vi "Get IBEE Results.vi"(8 "error in (no error)":errorcluster, 11 "niDTS BT INSTR TX in":refnum<class "niDTS BT INSTR TX.lvclass">) -> (0 "error out":errorcluster, 2 "IBE Results":T1, 3 "niDTS BT INSTR TX out":refnum<class "niDTS BT INSTR TX.lvclass">)   [LabVIEW 2015, in "niDTS BT.lvlib" / "niDTS BT INSTR TX.lvclass"]
uses:
  niDTS BT INSTR TX.lvclass
  Tests/Tx Test/Includes/niDTS BT Tx Test INC IBE Results.ctl
  niDTS BT INSTR TX.lvclass/niDTS BT INSTR TX.ctl
  RiviInstDriver/niRfsaBT/Objects/niRfsaBt.lvclass
  niDTS BT.lvlib
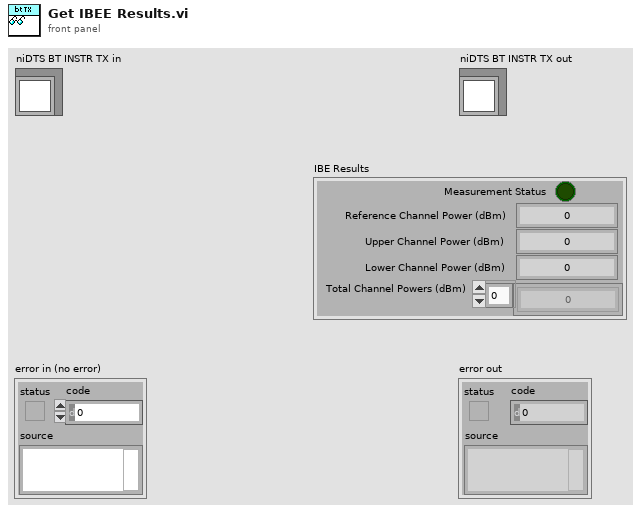
[diagram p1: front panel]
types:
  T1 = typedef "niDTS BT.lvlib/niDTS BT Tx Test INC IBE Results.ctl" = cluster{"Measurement Status":bool, "Reference Channel Power (dBm)":dbl, "Upper Channel Power (dBm)":dbl, "Lower Channel Power (dBm)":dbl, "Total Channel Powers (dBm)":dbl[]}
  T2 = cluster{"MeasurementStatus":enum16{"PASS", "FAIL"}, "ReferenceChannelPower":dbl, "UpperChannelTotalPower":dbl, "LowerChannelTotalPower":dbl, "TotalChannelPower":dbl[]}
  T3 = typedef "niRfsaBT.lvclass/niRfsaBT INC Handle.ctl" = refnum<data-value>
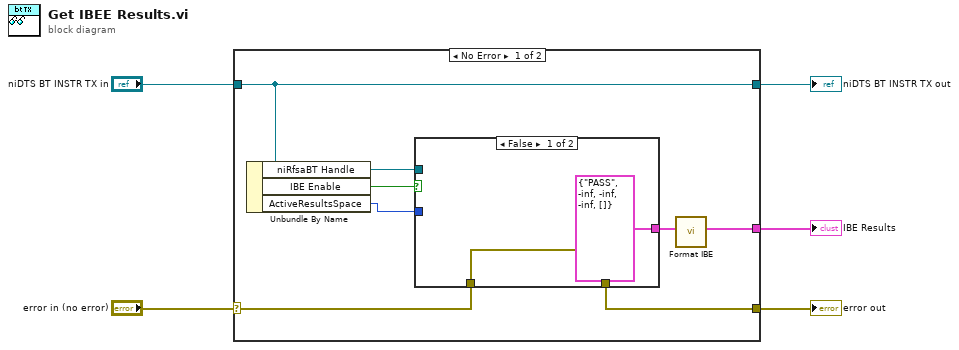
[diagram p0: block diagram]
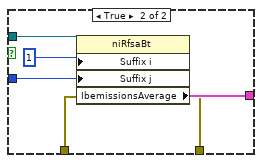
[diagram p2: hidden frame]
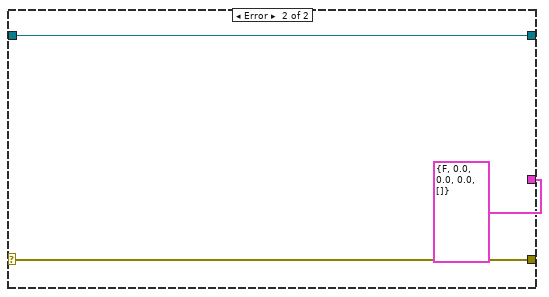
[diagram p3: hidden frame]
diagram:
  n1 = case shown="No Error" "error in (no error)" {
    selector: "error in (no error)" -> [w7 w23]
    tunnel: [w6 w23] -> w4
    tunnel: [w13 w24] -> w2
    tunnel: "niDTS BT INSTR TX in" -> [w13 w24]
    tunnel: [w9 T1 {"Measurement Status"=FALSE, "Reference Channel Power (dBm)"=0.0, "Upper Channel Power (dBm)"=0.0, "Lower Channel Power (dBm)"=0.0, "Total Channel Powers (dBm)"=[]} ("IBE Results")] -> w1
    frame No Error {
      n2 = Unbundle By Name(w13) -> ("niRfsaBT Handle"=w12:T3, "IBE Enable"=w11:bool, "ActiveResultsSpace"=w8:u8)
      n3 = case shown="False" w11 {
        tunnel: w12 -> [_ w21]
        tunnel: [T2 {"MeasurementStatus"=enum."PASS", "ReferenceChannelPower"=-inf, "UpperChannelTotalPower"=-inf, "LowerChannelTotalPower"=-inf, "TotalChannelPower"=[]} ("IBEMissionsi") w19] -> w10
        tunnel: w8 -> [_ w18]
        tunnel: w7 -> [w14 w17]
        tunnel: [w14 w16] -> w6
        frame False {
        }
        frame True {
          n4 = property class="niRfsaBt"(reference=w21, error in=w17, "Suffix i"=1 ("Active Channel:Suffix i"), "Suffix j"=w18) -> (error out=w16:errorcluster, "IbemissionsAverage"=w19:T2)  [unwired: 1 out]
        }
      }
      n5 = call "Format IBE.vi"("IBEMissionsion"=w10) -> ("IBE Results"=w9:T1)  [unwired: 10 in]
    }
    frame Error {
    }
  }
  "error out" <- w4
  "niDTS BT INSTR TX out" <- w2
  "IBE Results" <- w1
